vi "setFPGAReference.vi"(10 "FPGAReference":refnum<k20>, 11 "FPGATelemetry in":refnum<class "RTHealthAndStatus.lvclass">) -> (3 "FPGATelemetry out":refnum<class "RTHealthAndStatus.lvclass">)   [LabVIEW 2015]
uses:
  RTHealthAndStatus.lvclass
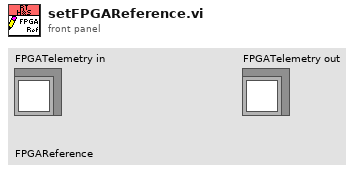
[diagram p1: front panel]
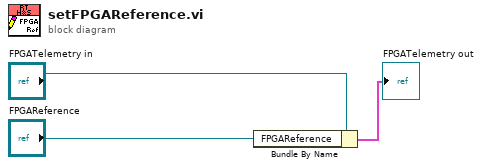
[diagram p0: block diagram]
diagram:
  n1 = Bundle By Name(cluster="FPGATelemetry in", "FPGAReference"="FPGAReference") -> (→"FPGATelemetry out":cluster{})
